vi "PDF Protokoll EPA1065_LeakCheck.vi"(8 "error in (no error)":errorcluster caption="Fehler (Eingang, kein Fehler)") -> (0 "error out":errorcluster caption="Fehler (Ausgang)")   [LabVIEW 2020, in "EPA 1065.lvlib" / "Dichtheitstest 1065-345.lvlib"]
uses:
  Dichtheitstest 1065-345.lvlib
  Versa Button.ctl
  VFS Button.ctl
  Aktion Protokolldaten_Leak check.ctl
  Aktion Leak Daten.ctl
  Sprachverwaltung/FGV Aktion Tabelle zerlegen.ctl
  <vilib>/Utility/miscctls.llb/LVRowAndColumnTypeDef.ctl
  <vilib>/Utility/miscctls.llb/LVPrintingMarginsTypeDef.ctl
  Allgemein/allgemeine Sub-VIs.lvlib
  Sprachverwaltung/Sprachverwaltung.lvlib
panel:
  in  "VFS button":T1
  in  "FAS button":T2
  out "EPA Konform":string
  out "Inner diameter \nHL to SP":sgl format="%#_5g"
  out "Length HL to SP":sgl format="%#_5g"
  out "Total volume VFS":sgl
  out "Length HL to VFS":sgl format="%#_5g"
  out "Inner diameter  \nHL to VFS":sgl format="%#_5g"
  out "Total volume versa":sgl caption="Total volume Versa"
  out "Heizleitung\nzum\nVFS":bool caption="Heated line\nto\nVFS"
  out "Heizleitung\nzur\nEntnahmestelle":bool caption="Heated Line\nto\nSampling point"
  out "VFS":bool
  out "Tabelle":string[][](table)
  # "Leak Check - EPA § 1065.345"
  # "mm"
  # "mm"
  # "mm³"
  # "mm"
  # "mm"
  # "mm³"
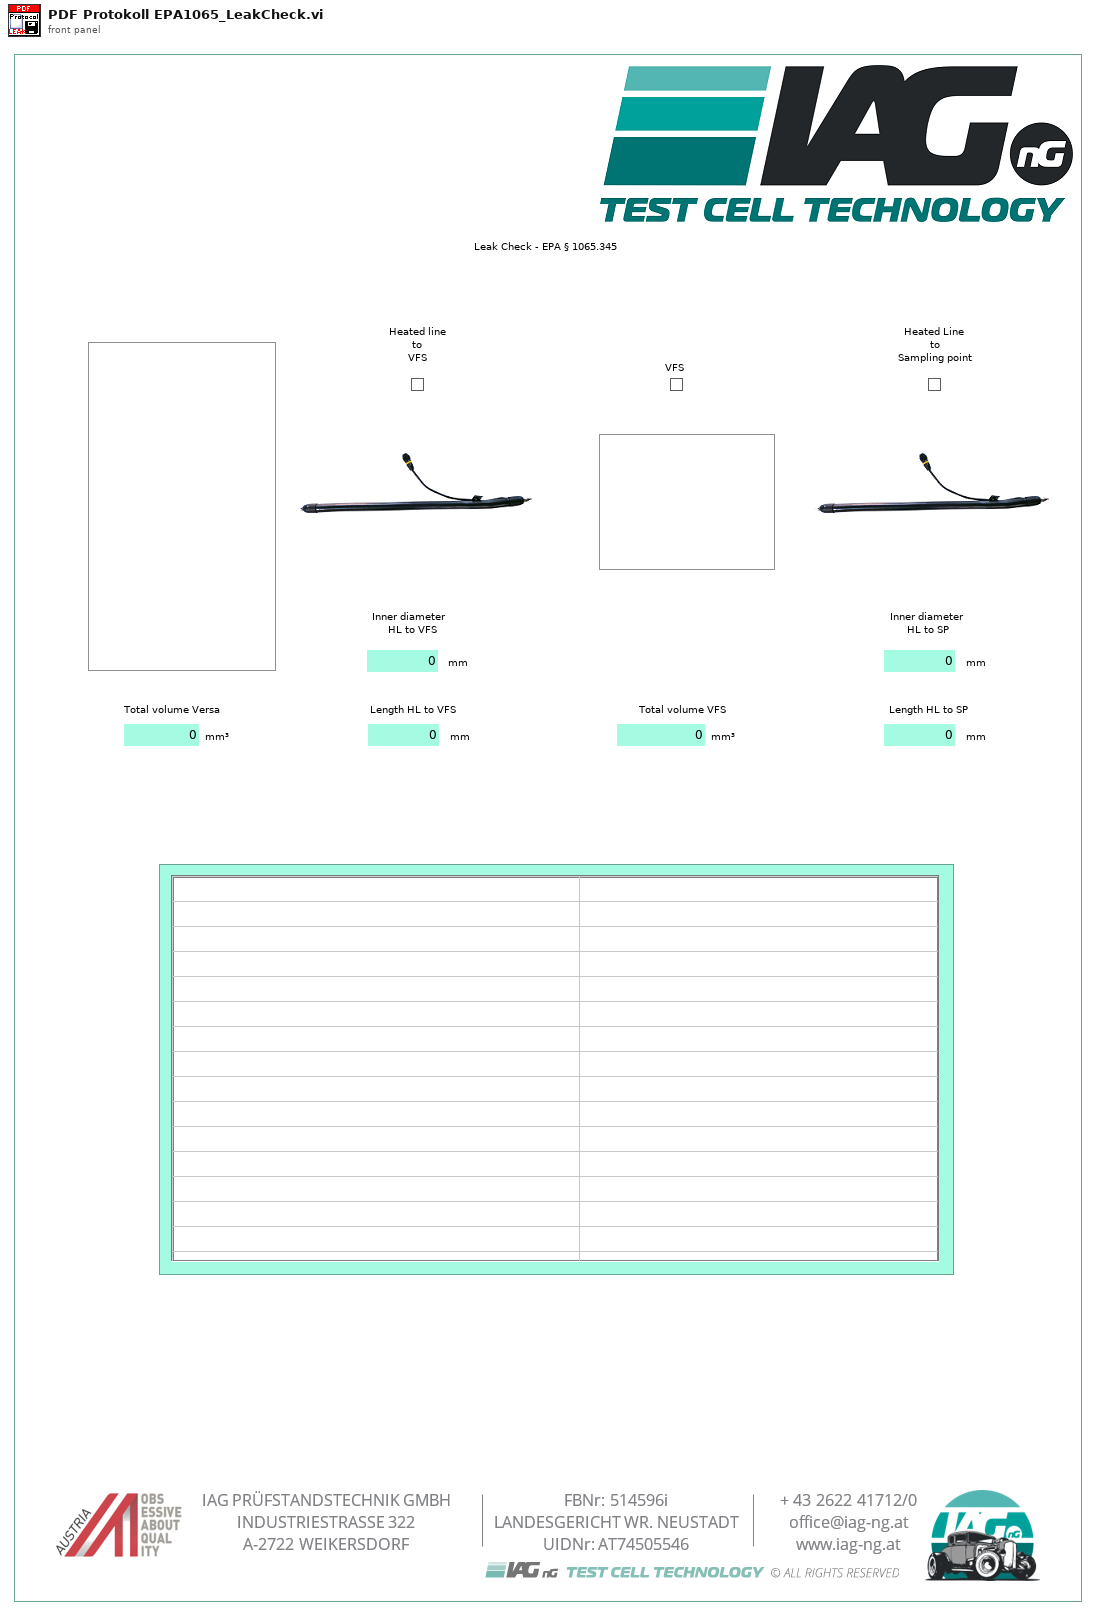
[diagram p1: front panel]
types:
  T1 = typedef "EPA 1065.lvlib/Dichtheitstest 1065-345.lvlib/VFS Button.ctl" = bool
  T2 = typedef "EPA 1065.lvlib/Dichtheitstest 1065-345.lvlib/Versa Button.ctl" = bool
  T3 = typedef "LVRowAndColumnTypeDef.ctl" = cluster{"Row":i32, "Column":i32}
  T4 = typedef "Sprachverwaltung.lvlib/FGV Aktion Tabelle zerlegen.ctl" = enum16{"laden", "vereinzeln", "speichern"}
  T5 = typedef "EPA 1065.lvlib/Dichtheitstest 1065-345.lvlib/Aktion Leak Daten.ctl" = enum16{"lesen", "laden", "speichern", "Volumen", "berechnen", "Leak check aktiv", "Leak Zustand", "Pfad", "Pfad speichern"}
  T6 = typedef "EPA 1065.lvlib/Dichtheitstest 1065-345.lvlib/Aktion Protokolldaten_Leak check.ctl" = enum16{"lesen", "Zeitstempel", "Bearbeiter", "Daten", "Auswertung", "löschen"}
  T7 = typedef "LVPrintingMarginsTypeDef.ctl" = cluster{"Top":sgl, "Left":sgl, "Bottom":sgl, "Right":sgl, "Measurement System":enum8{"Inches", "cm"}}
  T8 = enum32{"Portrait", "Landscape", "Rotated Portrait", "Rotated Landscape"}
  T9 = typedef "EPA 1065.lvlib/Dichtheitstest 1065-345.lvlib/Gesamtvolumen.ctl" = cluster{"FAS":sgl, "d von HL zu VFS":sgl, "l von HL zu VFS":sgl, "VFS":sgl, "d von HL zu SP":sgl, "l von HL zu SP":sgl, "Heizleitung zum VFS":bool, "VFS a":bool, "Heizleitung zur Entnahmestelle":bool, "Gesamtes Volumen":sgl, "LeakValve":u16, "Einheit":enum16{"mol/s", "mbar"}}
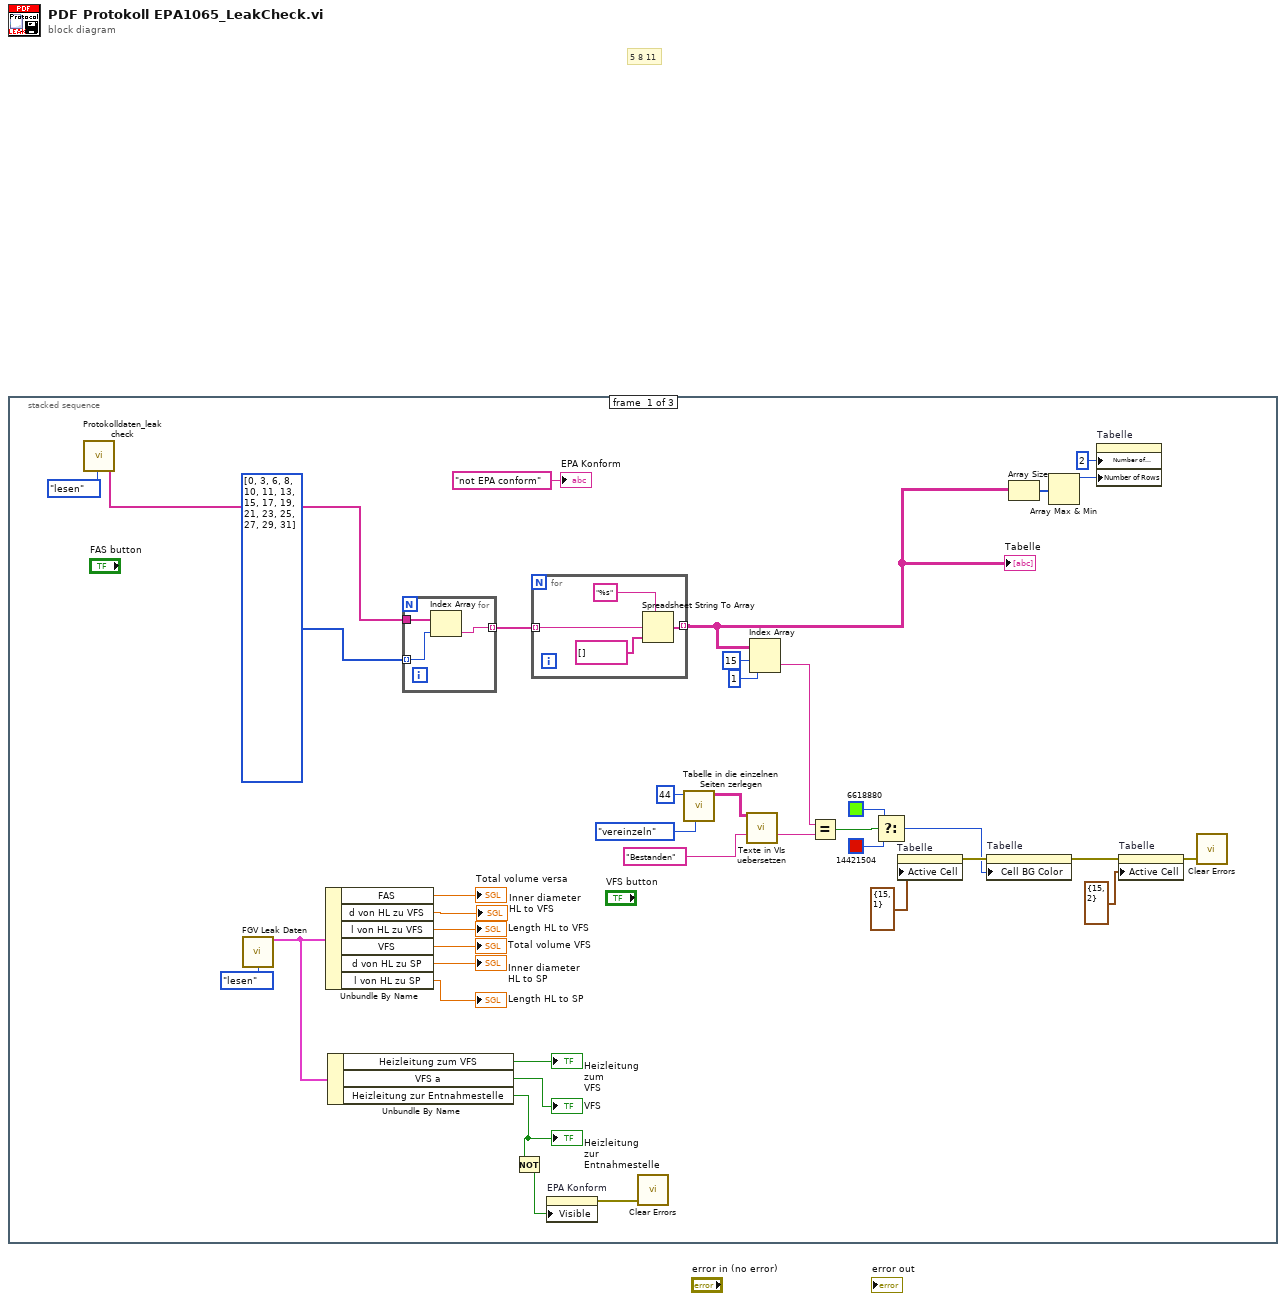
[diagram p0: block diagram]
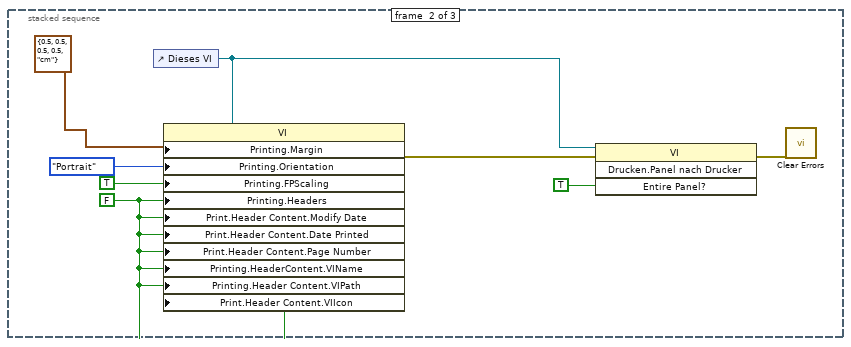
[diagram p2: hidden frame]
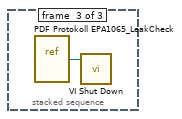
[diagram p3: hidden frame]
diagram:
  # "5 8 11"
  n1 = stacked-sequence {
    frame #0 {
      n2 = call "Protokolldaten_leak check.vi"("Aktion"=Aktion_Protokolldaten_Leak_check."lesen") -> ("Auswertung"=w35:string[])  [unwired: 23 in, 3 out]
      n3 = call "FGV Leak Daten.vi"("Aktion"=Aktion_Leak_Daten."lesen") -> ("Gesamtvolumen"=w33:T9)  [unwired: 10 in, 4 out]
      n4 = Unbundle By Name(w33) -> ("FAS"=→"Total volume versa":sgl, "d von HL zu VFS"=→"Inner diameter  \nHL to VFS":sgl, "l von HL zu VFS"=→"Length HL to VFS":sgl, "VFS"=→"Total volume VFS":sgl, "d von HL zu SP"=→"Inner diameter \nHL to SP":sgl, "l von HL zu SP"=→"Length HL to SP":sgl)
      n5 = Unbundle By Name(w33) -> ("Heizleitung zum VFS"=→"Heizleitung\nzum\nVFS":bool, "VFS a"=→"VFS":bool, "Heizleitung zur Entnahmestelle"=w2:bool)
      "Heizleitung\nzur\nEntnahmestelle" <- w2
      n6 = for {
        tunnel: w35 -> [w46]
        tunnel: i32[] [0, 3, 6, 8, 10, 11, 13, 15, 17, 19, 21, 23, 25, 27, 29, 31] -> [w45] mode=indexing
        tunnel: [w44] -> w7 mode=indexing
        n7 = Index Array(array=w46, index=w45) -> (element=w44:string)
      }
      n8 = Not(x=w2) -> (.not. x?=w1:bool)
      n9 = for {
        tunnel: [w42] -> w28 mode=indexing
        tunnel: w7 -> [w40] mode=indexing
        n10 = Spreadsheet String To Array(format string="%s" ("Format-String"), spreadsheet string=w40, array type (2D Dbl)=string[] []) -> (array=w42:string[])  [unwired: 1 in]
      }
      "Tabelle" <- w28
      n11 = property on="EPA Konform" class="Str"("Visible"=w1) -> (error out=w3:errorcluster)  [unwired: 2 in, 1 out]
      n12 = call <vilib>:"Clear Errors.vi"("error in (no error)"=w3) -> ()  [unwired: 5 in, 2 out]
      n13 = call "Tabelle in die einzelnen Seiten zerlegen.vi"("Aktion"=FGV_Aktion_Tabelle_zerlegen."vereinzeln", "Index (Seite)"=44) -> ("Sprachliste"=w24:string[][])  [unwired: 7 in, 2 out]
      n14 = call "Texte in VIs uebersetzen.vi"("Sprachliste"=w24, "String zum Übersetzen"="Bestanden" ("Element")) -> ("String zum Übersetzen"=w27:string)  [unwired: 9 in, 4 out]
      n15 = Index Array(array=w28, index (row)=15 ("Index (Zeile)"), index (col)=1 ("Deaktivierter Index (Spalte)")) -> (element=w22:string)
      n16 = Equal?(x=w22, y=w27) -> (x = y?=w21:bool)
      n17 = Select(t=u32 6618880, s=w21, f=u32 14421504) -> (s? t:f=w18:u32)
      n18 = property on="Tabelle" class="Tbl (strikt)"("Active Cell"=T3 {"Row"=15, "Column"=1} ("Aktive Zelle:Aktive Zelle")) -> (error out=w19:errorcluster)  [unwired: 2 in, 1 out]
      n19 = property on="Tabelle" class="Tbl (strikt)"(error in=w19, "Cell BG Color"=w18) -> (error out=w17:errorcluster)  [unwired: 1 in, 1 out]
      n20 = Array Size(array=w28) -> (size(s)=w38:i32[])
      n21 = Array Max & Min(array=w38) -> (max value=w37:i32)  [unwired: 3 out]
      n22 = property on="Tabelle" class="Tbl (strikt)"("Number of Columns"=u32 2 ("Spaltenanzahl"), "Number of Rows"=w37) -> ()  [unwired: 2 in, 2 out]
      n23 = property on="Tabelle" class="Tbl (strikt)"(error in=w17, "Active Cell"=T3 {"Row"=15, "Column"=2} ("Aktive Zelle:Aktive Zelle")) -> (error out=w15:errorcluster)  [unwired: 1 in, 1 out]
      n24 = call <vilib>:"Clear Errors.vi"("error in (no error)"=w15) -> ()  [unwired: 5 in, 2 out]
      "EPA Konform" <- "not EPA conform" ("EPA Konform")
    }
    frame #1 {
      w50 = FALSE ("Drucken:Kopfzeilen?")
      n25 = control-ref of="Dieses VI"() -> (w47:refnum<vi>)
      n26 = property class="VI"(reference=w47, "Printing.Margin"=T7 {"Top"=0.5, "Left"=0.5, "Bottom"=0.5, "Right"=0.5, "Measurement System"=enum."cm"} ("Drucken:Ränder"), "Printing.Orientation"=T8."Portrait" ("Drucken:Seitenausrichtung"), "Printing.FPScaling"=TRUE ("Drucken:Frontpanel-Skalierung?"), "Printing.Headers"=w50, "Print.Header Content.Modify Date"=w50, "Print.Header Content.Date Printed"=w50, "Print.Header Content.Page Number"=w50, "Printing.HeaderContent.VIName"=w50, "Printing.Header Content.VIPath"=w50, "Print.Header Content.VIIcon"=w50) -> (error out=w54:errorcluster)  [unwired: 1 in, 1 out]
      n27 = invoke class="VI" method="Drucken.Panel nach Drucker"(reference=w47, error in=w54, "Entire Panel?"=TRUE ("Abschnittskopfzeilen?")) -> (error out=w48:errorcluster)  [unwired: 1 in, 3 out]
      n28 = call <vilib>:"Clear Errors.vi"("error in (no error)"=w48) -> ()  [unwired: 5 in, 2 out]
    }
    frame #2 {
      n29 = vi-ref "PDF Protokoll EPA1065_LeakCheck.vi"() -> (w55:refnum<vi>)
      n30 = call "VI Shut Down.vi"("VI Referenz"=w55) -> ()  [unwired: 11 in]
    }
  }
